vi "vision testing.vi"() -> ()   [LabVIEW 2012]
panel:
  in  "Tab Control":T1(tab)
  out "No":bool
  in  "Targeted Goal":dbl[](array[numeric])
  out "Yes":bool
  in  "Start":bool
  in  "Use VI Dir?":bool
  in  "Differnt or Ordered?":T2(tab)
  in  "Names / Paths":string[](array[string])
  in  "Width 0-6":dbl
  in  "End Number":dbl
  in  "Start Number":dbl
  in  "File Type":string(combo)=".bmp"
  in  "Prefix":string
  in  "File Name":string
  in  "Root Path":path
  in  "stop":bool
  out "Picture File Path":path[](array[path])
  out "Distance":string[](array[string])
  out "Auto Rotation":dbl[](array[numeric])
  out "Highlight Array":dbl[][][](array[numeric])
  out "Class Array":dbl[][][](array[numeric])
  out "Class Transposed":dbl[][][](array[numeric])
  out "Cases Array":dbl[][][](array[numeric])
  out "Selected Goal Subarray":dbl[][](array[numeric])
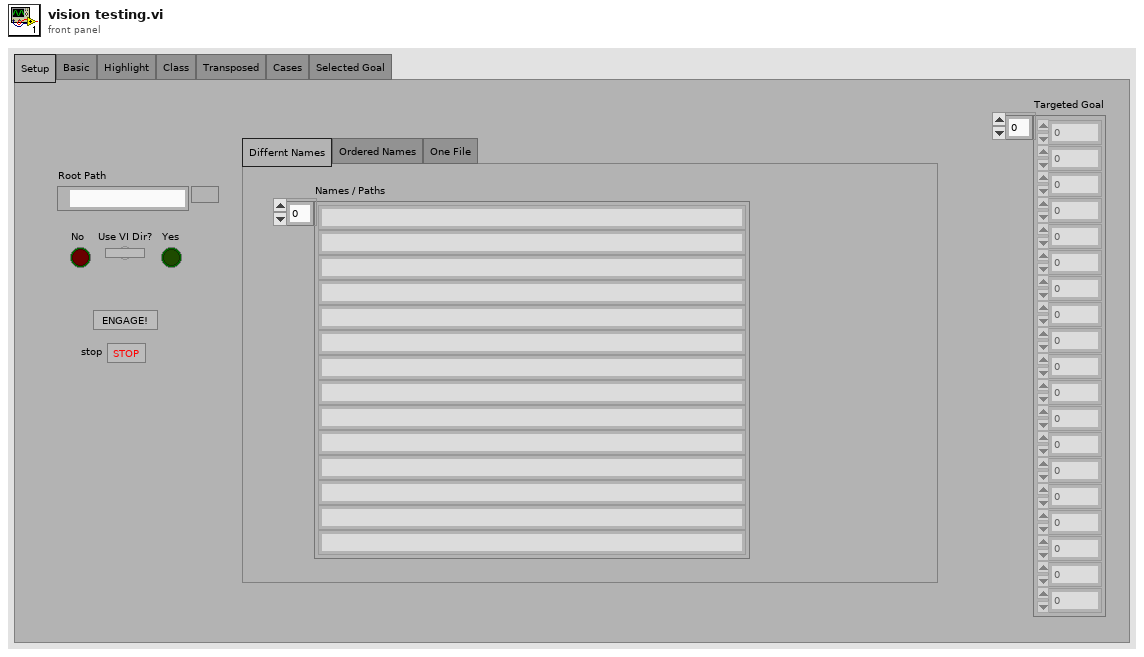
[diagram p1: front panel]
types:
  T1 = enum32{"Setup", "Basic", "Highlight", "Class", "Transposed", "Cases", "Selected Goal"}
  T2 = enum32{"Differnt Names", "Ordered Names", "One File"}
  T3 = typedef "Image Type" = u32
  T4 = typedef "IMAQ Image.ctl" = refnum<image>
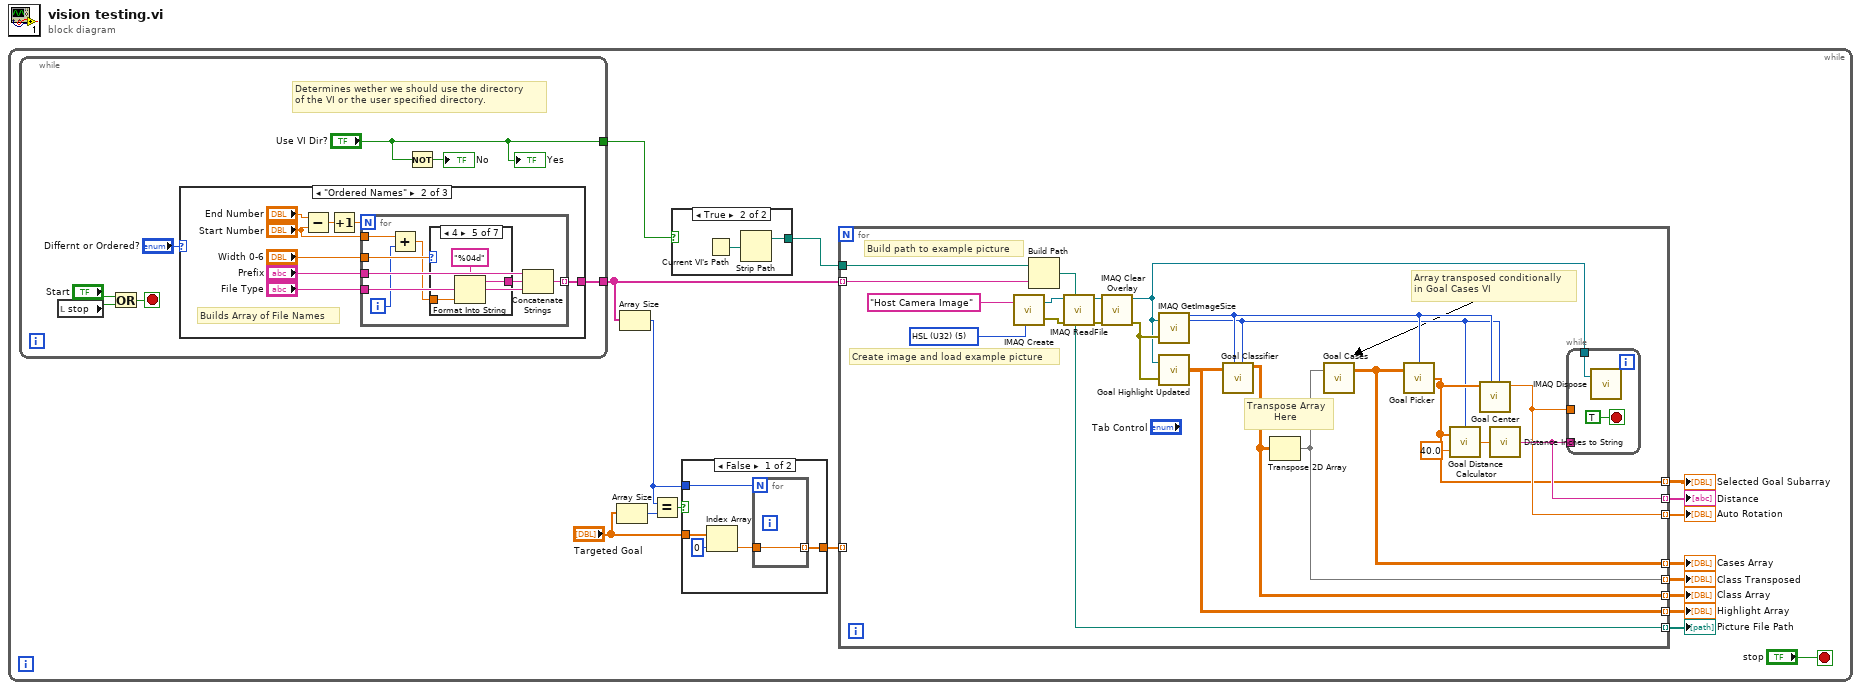
[diagram p0: block diagram]
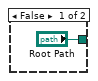
[diagram p3: hidden frame]
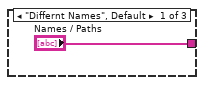
[diagram p4: hidden frame]
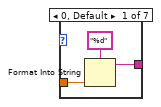
[diagram p5: hidden frame]
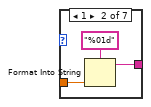
[diagram p6: hidden frame]
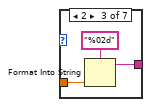
[diagram p7: hidden frame]
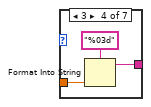
[diagram p8: hidden frame]
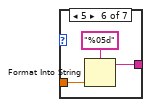
[diagram p9: hidden frame]
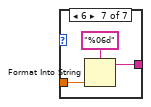
[diagram p10: hidden frame]
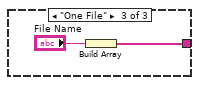
[diagram p11: hidden frame]
diagram:
  n1 = while {
    stop <- "stop" stop-if-true
    n2 = while {
      tunnel: ["Use VI Dir?"] -> w17
      tunnel: [w57] -> w16
      stop <- w54 stop-if-true
      # "Determines wether we should use the directory \nof the VI or the user specified directory."
      n3 = local read "stop"() -> (w52:bool)
      n4 = Or(x="Start", y=w52) -> (x .or. y?=w54:bool)
      n5 = case shown="\"Ordered Names\"" "Differnt or Ordered?" {
        tunnel: ["Names / Paths" w62 w97] -> w57
        frame "Differnt Names", Default {
        }
        frame "Ordered Names" {
          # "Builds Array of File Names"
          n6 = Subtract(x="End Number", y="Start Number") -> (x-y=w61:dbl)
          n7 = Increment(x=w61) -> (x+1=w60:dbl)
          n8 = for {
            N: w60 -> [_]
            tunnel: "Start Number" -> [w74]
            tunnel: "Width 0-6" -> [w75]
            tunnel: "Prefix" -> [w73]
            tunnel: "File Type" -> [w72]
            tunnel: [w71] -> w62 mode=indexing
            i -> [w68]
            n9 = Add(x=w74, y=w68) -> (x+y=w69:dbl)
            n10 = case shown="4" w75 {
              tunnel: [w77 w80 w83 w86 w89 w92 w95] -> w70
              tunnel: w69 -> [w76 w79 w82 w85 w88 w91 w94]
              frame 0, Default {
                n11 = Format Into String(format string="%d", w76) -> (resulting string=w77:string)  [unwired: 2 in, 1 out]
              }
              frame 1 {
                n12 = Format Into String(format string="%01d", w79) -> (resulting string=w80:string)  [unwired: 2 in, 1 out]
              }
              frame 2 {
                n13 = Format Into String(format string="%02d", w82) -> (resulting string=w83:string)  [unwired: 2 in, 1 out]
              }
              frame 3 {
                n14 = Format Into String(format string="%03d", w85) -> (resulting string=w86:string)  [unwired: 2 in, 1 out]
              }
              frame 4 {
                n15 = Format Into String(format string="%04d", w88) -> (resulting string=w89:string)  [unwired: 2 in, 1 out]
              }
              frame 5 {
                n16 = Format Into String(format string="%05d", w91) -> (resulting string=w92:string)  [unwired: 2 in, 1 out]
              }
              frame 6 {
                n17 = Format Into String(format string="%06d", w94) -> (resulting string=w95:string)  [unwired: 2 in, 1 out]
              }
            }
            n18 = Concatenate Strings(w73, w70, w72) -> (w71:string)
          }
        }
        frame "One File" {
          n19 = Build Array("File Name") -> (w97:string[])
        }
      }
      n20 = Not(x="Use VI Dir?") -> (.not. x?=→"No":bool)
      "Yes" <- "Use VI Dir?"
    }
    n21 = Array Size(array="Targeted Goal") -> (size(s)=w12:i32)
    n22 = Array Size(array=w16) -> (size(s)=w11:i32)
    n23 = Equal?(x=w11, y=w12) -> (x = y?=w13:bool)
    n24 = case shown="True" w17 {
      tunnel: ["Root Path" w26] -> w15
      frame False {
      }
      frame True {
        n25 = Current VI's Path() -> (path=w27:path)
        n26 = Strip Path(path=w27) -> (stripped path=w26:path)  [unwired: 1 out]
      }
    }
    n27 = case shown="False" w13 {
      tunnel: [w22 w24] -> w14
      tunnel: w11 -> [w21 _]
      tunnel: "Targeted Goal" -> [w20 w24]
      frame False {
        n28 = Index Array(array=w20, index=0) -> (element=w18:dbl)
        n29 = for {
          N: w21 -> [_]
          tunnel: [w23] -> w22 mode=indexing
          tunnel: w18 -> [w23]
        }
      }
      frame True {
      }
    }
    n30 = for {
      tunnel: w15 -> [w47]
      tunnel: w16 -> [w46] mode=indexing
      tunnel: [w38] -> w9 mode=indexing
      tunnel: [w37] -> w6 mode=indexing
      tunnel: [w36] -> w5 mode=indexing
      tunnel: [w35] -> w4 mode=indexing
      tunnel: [w49] -> w3 mode=indexing
      tunnel: [w33] -> w7 mode=indexing
      tunnel: [w34] -> w8 mode=indexing
      tunnel: w14 -> [_] mode=indexing
      tunnel: [w31] -> w1 mode=indexing
      w44 = T3 5 items=["Grayscale (U8)", "Grayscale (I16)", "Grayscale (SGL)", "Complex (CSG)", "RGB (U32)", "HSL (U32)", "RGB (U64)"] ("Image Type")
      # "Create image and load example picture"
      # "Array transposed conditionally\nin Goal Cases VI"
      # "Transpose Array\n         Here"
      # "Build path to example picture"
      n31 = call "IMAQ Create"("Image Name"="Host Camera Image", "Image Type"=w44) -> ("New Image"=w43:T4, "error out"=w42:errorcluster)  [unwired: 2 in, 1 out]
      n32 = Build Path(base path=w47, name or relative path=w46) -> (appended path=w38:path)
      n33 = call "IMAQ ReadFile"("File Path"=w38, "error in (no error)"=w42, "Image"=w43) -> ("error out"=w41:errorcluster, "Image Out"=w48:T4)  [unwired: 4 in, 3 out]
      n34 = call "IMAQ Clear Overlay"("error in (no error)"=w41, "Image"=w48) -> ("error out"=w40:errorcluster, "Image Out"=w39:T4)  [unwired: 1 in, 7 out]
      n35 = call "IMAQ GetImageSize"("Image"=w39, "error in (no error)"=w40) -> ("Y Resolution"=w29:i32, "X Resolution"=w32:i32)  [unwired: 2 in, 1 out]
      n36 = call "Goal Highlight Updated.vi"("Image In"=w39, "error in"=w40) -> ("Particle Measurements (Pixels)"=w37:dbl[][])  [unwired: 2 out]
      n37 = call "Goal Classifier.vi"("ResolutionY"=w29, "ResolutionX"=w32, "InArray"=w37) -> ("OutArray"=w36:dbl[][])  [unwired: 8 in]
      n38 = Transpose 2D Array(2D array=w36) -> (transposed array=w35:dbl[][])
      n39 = call "Goal Cases.vi"("InArray"=w35) -> ("OutArray"=w49:dbl[][])  [unwired: 1 in, 1 out]
      n40 = call "Goal Picker.vi"("ResolutionX"=w32, "InArray"=w49) -> ("SelectedGoalSubarray"=w31:dbl[])  [unwired: 1 in]
      n41 = call "Goal Distance Calculator.vi"("ResolutionY"=w29, "Theda"=40.0, "InArray"=w31) -> ("DistanceOut"=w28:dbl)
      n42 = call "Goal Center.vi"("ResolutionY"=w29, "ResolutionX"=w32, "SelectedGoalSubarray"=w31) -> ("PsuedoJoystickOutRotation"=w33:dbl)  [unwired: 8 in]
      n43 = call "Distance Inches to String.vi"("Distance Inches"=w28) -> ("Distance String"=w34:string)
      n44 = while {
        tunnel: w39 -> [w51]
        tunnel: w34 -> [_]
        tunnel: w33 -> [_]
        stop <- TRUE stop-if-true
        n45 = call "IMAQ Dispose"("Image"=w51) -> ()  [unwired: 5 in, 1 out]
      }
    }
    "Distance" <- w8
    "Auto Rotation" <- w7
    "Picture File Path" <- w9
    "Highlight Array" <- w6
    "Class Array" <- w5
    "Class Transposed" <- w4
    "Cases Array" <- w3
    "Selected Goal Subarray" <- w1
  }
